vi "Throwing Arm.vi"() -> ()   [LabVIEW 2014]
uses:
  <vilib>/National Instruments/NI Dynamixel API/Dynamixel Driver/Controls/Baud Rate Selector.ctl
  <vilib>/National Instruments/NI Dynamixel API/Dynamixel Driver/Controls/Joints.ctl
  <vilib>/National Instruments/NI Dynamixel API/Dynamixel Driver/Controls/Joint.ctl
  <vilib>/National Instruments/NI Dynamixel API/Dynamixel Driver/Dynamixel Driver Code.lvlib
panel:
  in  "JOSH SWING":dbl[][](array[numeric])=[[2000.0, 150.0, 200.0, 0.0, 60.0, 230.0, 0.0, 223.0], [400.0, 200.0, 270.0, 0.0, 60.0, 230.0, 0.0, 223.0], [400.0, 0.0, 30.0, 0.0, 60.0, 230.0, 0.0, 223.0], [750.0, 220.0, 260.0, 0.0, 60.0, 230.0, 0.0, 223.0], [400.0, 220.0, 260.0, 0.0, 60.0, 230.0, 0.0, 150.0], [600.0, 115.0, 70.0, 0.0, 60.0, 115.0, 0.0, 223.0], [200.0, 115.0, 70.0, 0.0, 60.0, 115.0, 0.0, 223.0], [500.0, 115.0, 70.0, 0.0, 60.0, 115.0, 0.0, 223.0]]
  in  "SWING":dbl[][](array[numeric])=[[400.0, 115.0, 70.0, 0.0, 20.0, 250.0, 0.0, 223.0], [400.0, 0.0, 10.0, 0.0, 120.0, 80.0, 0.0, 223.0], [700.0, 175.0, 70.0, 0.0, 20.0, 250.0, 0.0, 223.0], [500.0, 0.0, 10.0, 0.0, 120.0, 80.0, 0.0, 223.0], [50.0, 350.0, 10.0, 0.0, 120.0, 80.0, 0.0, 223.0], [600.0, 220.0, 260.0, 0.0, 30.0, 230.0, 0.0, 223.0], [200.0, 220.0, 260.0, 0.0, 30.0, 230.0, 0.0, 150.0], [500.0, 115.0, 70.0, 0.0, 60.0, 115.0, 0.0, 223.0]]
  in  "Hard Throw  2":dbl[][](array[numeric])=[[400.0, 115.0, 70.0, 0.0, 20.0, 250.0, 0.0, 223.0], [400.0, 0.0, 10.0, 0.0, 120.0, 80.0, 0.0, 223.0], [700.0, 175.0, 70.0, 0.0, 20.0, 250.0, 0.0, 223.0], [500.0, 0.0, 10.0, 0.0, 120.0, 80.0, 0.0, 223.0], [50.0, 350.0, 10.0, 0.0, 120.0, 80.0, 0.0, 223.0], [600.0, 220.0, 260.0, 0.0, 30.0, 230.0, 0.0, 223.0], [200.0, 220.0, 260.0, 0.0, 30.0, 230.0, 0.0, 150.0], [500.0, 115.0, 70.0, 0.0, 60.0, 115.0, 0.0, 223.0]]
  in  "Gripper\nOpen/Close":bool
  in  "THROW!":bool
  in  "Standard Throw":dbl[][](array[numeric])=[[400.0, 115.0, 70.0, 0.0, 20.0, 250.0, 0.0, 223.0], [400.0, 0.0, 10.0, 0.0, 120.0, 80.0, 0.0, 223.0], [700.0, 175.0, 70.0, 0.0, 20.0, 250.0, 0.0, 223.0], [500.0, 0.0, 10.0, 0.0, 120.0, 80.0, 0.0, 223.0], [50.0, 350.0, 10.0, 0.0, 120.0, 80.0, 0.0, 223.0], [600.0, 220.0, 260.0, 0.0, 30.0, 230.0, 0.0, 223.0], [200.0, 220.0, 260.0, 0.0, 30.0, 230.0, 0.0, 150.0], [500.0, 115.0, 70.0, 0.0, 60.0, 115.0, 0.0, 223.0]]
  out "Elbow":dbl(knob) scale=0.0..300.0
  out "Shoulder Angle":dbl(knob) scale=0.0..300.0
  out "All End Positions":T1 {"Goal Position (Degrees)" scale=0.0..300.0}
  in  "VISA Refnum in":refnum<visa-resource-name>="ASRL1::INSTR"
  in  "Baud Rate":T3
  in  "File Path Control":path=path "/Macintosh HD/Users/joshuasullivan/Dropbox/ROCO504/Showcase/RobotTest.ini"
  in  "Stop Button":bool
  # "Time"
  # "Servo1"
  # "Servo2"
  # "Shoulder"
  # "Servo4"
  # "Servo5"
  # "Elbow"
  # "Servo7"
  # "Elbow bend up"
  # "Move whole arm back"
  # "Whole arm forwards w/ elbow swing"
  # "Whole arm back"
  # "Shoulder build up tension"
  # "Arm forwards closed gripper"
  # "Arm forwards open gripper"
  # "Return and wait"
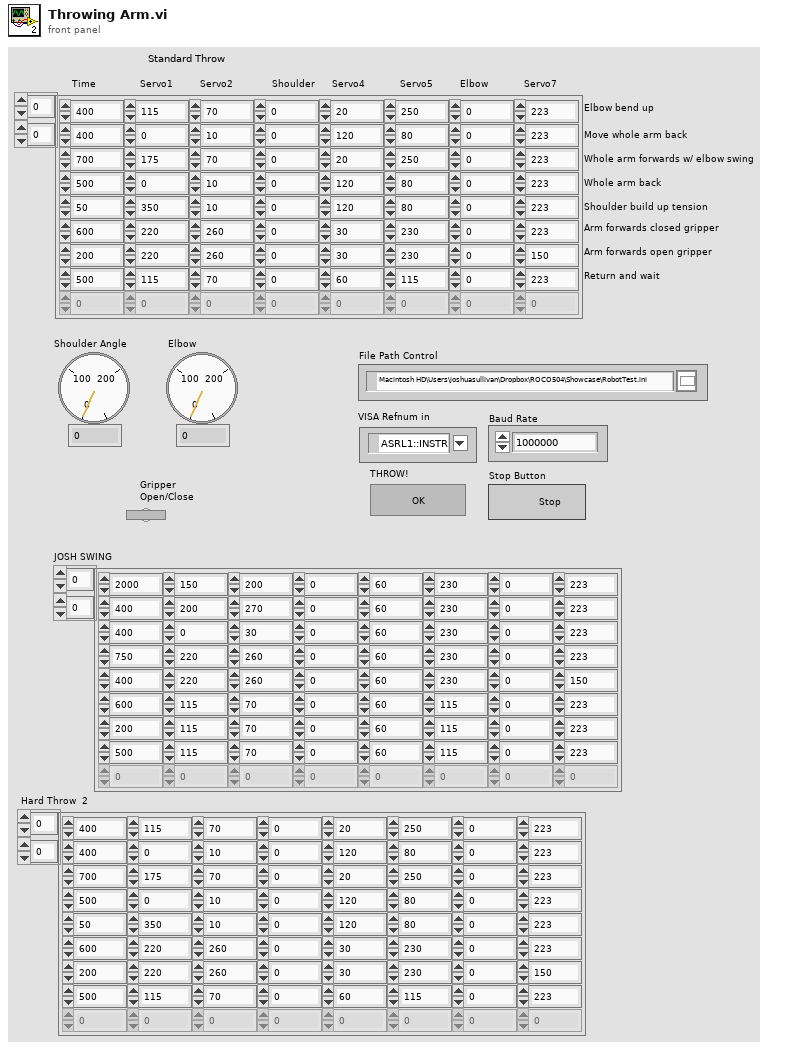
[diagram p1: front panel]
types:
  T1 = typedef "Dynamixel Driver Code.lvlib/Joints.ctl" = T2[]
  T2 = typedef "Dynamixel Driver Code.lvlib/Joint.ctl" = cluster{"Joint ID":dbl, "Goal Position (Degrees)":dbl}
  T3 = typedef "Dynamixel Driver Code.lvlib/Baud Rate Selector.ctl" = enum16{"1000000", "57600"}
  T4 = typedef "Dynamixel Driver Code.lvlib/Dynamixel Data.ctl" = T5[]
  T5 = typedef "Dynamixel Driver Code.lvlib/Single Dynamixel.ctl" = cluster{"ID":u8, "Speed":u16, "CW Margin/D":u8, "CCW Margin/I":u8, "CW Slope/P":u8, "CCW Slope/Accl":u8, "Punch":u16, "Joint":u8, "Max Position (Deg)":u16, "Min Position (Deg)":u16, "Torque Limit":u16, "Motor Type":T6, "Motor Model":T7, "Orientation":T8, "Sync Cable":T9}
  T6 = typedef "Dynamixel Driver Code.lvlib/Master Slave.ctl" = enum16{"Master", "Slave", "Sync"}
  T7 = typedef "Dynamixel Driver Code.lvlib/Motor Model.ctl" = enum16{"AX/DX/RX", "MX", "EX-106+"}
  T8 = typedef "Dynamixel Driver Code.lvlib/Orientation.ctl" = enum16{"Single", "Paired - Opposite", "Paired", "Same ID"}
  T9 = typedef "Dynamixel Driver Code.lvlib/Sync Cable.ctl" = enum16{"No", "Yes"}
  T10 = typedef "Dynamixel Driver Code.lvlib/Robot Session.ctl" = cluster{"VISA Resource":refnum<visa-resource-name>, "Dynamixel Data":T4}
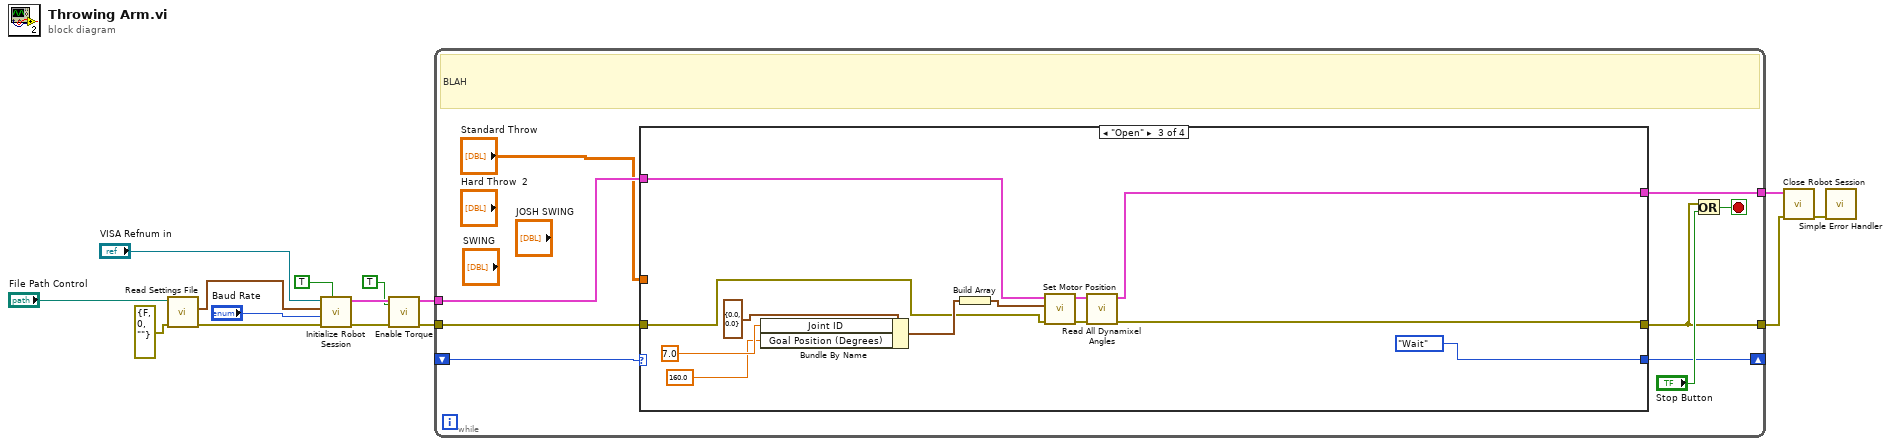
[diagram p0: block diagram]
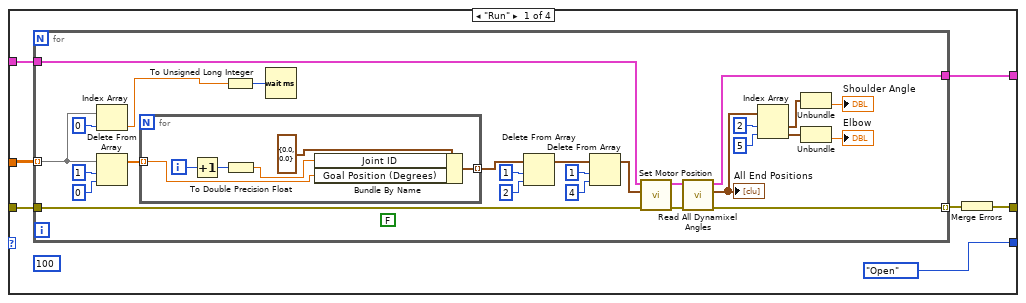
[diagram p2: hidden frame]
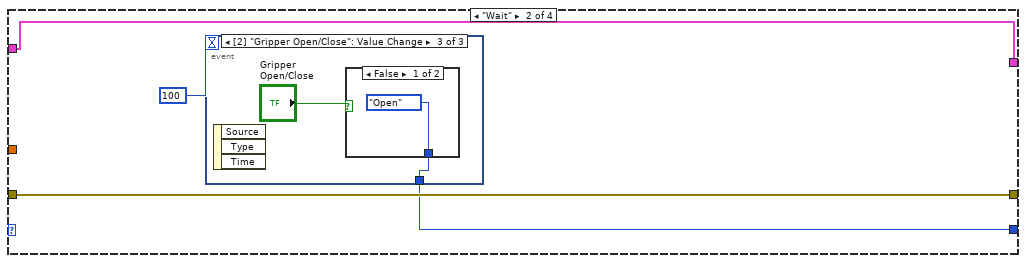
[diagram p3: hidden frame]
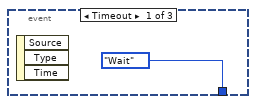
[diagram p4: hidden frame]
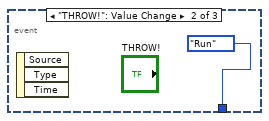
[diagram p5: hidden frame]
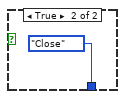
[diagram p6: hidden frame]
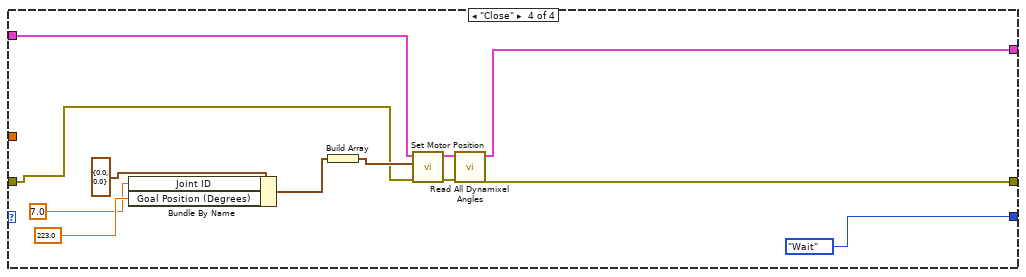
[diagram p7: hidden frame]
diagram:
  n1 = call <vilib>:"Read Settings File.vi"("error in (no error)"=errorcluster {"status"=FALSE, "code"=0, "source"=""} ("error constant"), "file path (dialog if empty)"="File Path Control") -> ("error out"=w14:errorcluster, "Dynamixel Data"=w7:T4)  [unwired: 8 in]
  n2 = call <vilib>:"Initialize Robot Session.vi"("Configure"=TRUE, "error in"=w14, "Baud Rate"="Baud Rate", "Initialization"=w7, "VISA Refnum in"="VISA Refnum in") -> ("error out"=w11:errorcluster, "Robot Session"=w12:T10)  [unwired: 5 in]
  n3 = call <vilib>:"Enable Torque.vi"("Set Goal Position to Current Position before Enable"=TRUE, "error in (no error)"=w11, "Robot Session In"=w12) -> ("error out"=w8:errorcluster, "Robot Session Out"=w10:T10)  [unwired: 6 in, 1 out]
  n4 = while {
    tunnel: w10 -> [w24]
    tunnel: w8 -> [w23]
    tunnel: [w22] -> w3
    tunnel: [w17] -> w2
    shift-right: [w19] -> _
    shift-left: _ -> [w18]
    stop <- w20 stop-if-true
    # "BLAH"
    n5 = case shown="\"Open\"" w18 {
      tunnel: w24 -> [w31 w68 w77 w91]
      tunnel: w23 -> [w30 w67 w76 w88]
      tunnel: [w29 w68 w79 w90] -> w22
      tunnel: [w26 w67 w78 w89] -> w17
      tunnel: "Standard Throw" -> [w28 _ _ _]
      tunnel: [enum16{"Close", "Open", "Wait", "Run"}."Open" w66 enum16{"Close", "Open", "Wait", "Run"}."Wait" enum16{"Close", "Open", "Wait", "Run"}."Wait"] -> w19
      frame "Run" {
        (unwired) 100
        n6 = for {
          tunnel: w28 -> [w54] mode=indexing
          tunnel: w31 -> [w43]
          tunnel: [w42] -> w29
          tunnel: [w41] -> w27 mode=indexing
          tunnel: w30 -> [w40]
          (unwired) FALSE ("stop")
          n7 = Index Array(array=w54, index=0 ("length")) -> (element=w32:dbl)
          n8 = Delete From Array(array=w54, length=1, index=0) -> (array with subset deleted=w55:dbl[])  [unwired: 1 out]
          n9 = for {
            tunnel: w55 -> [w59] mode=indexing
            tunnel: [w60] -> w39 mode=indexing
            i -> [w63]
            n10 = Increment(x=w63) -> (x+1=w62:i32)
            n11 = To Double Precision Float(number=w62) -> (double precision float=w61:dbl)
            n12 = Bundle By Name(cluster=T2 {"Joint ID"=0.0, "Goal Position (Degrees)"=0.0} ("Joint"), "Joint ID"=w61, "Goal Position (Degrees)"=w59) -> (w60:T2)
          }
          n13 = To Unsigned Long Integer(number=w32) -> (unsigned 32bit integer=w53:u32)
          n14 = Wait (ms)(milliseconds to wait=w53) -> ()  [unwired: 1 out]
          n15 = Delete From Array(array=w39, length=1, index=2 ("length")) -> (array with subset deleted=w36:T2[])  [unwired: 1 out]
          n16 = Delete From Array(array=w36, length=1, index=4) -> (array with subset deleted=w35:T2[])  [unwired: 1 out]
          n17 = call <vilib>:"Set Motor Position.vi"("error in (no error)"=w40, "Joints"=w35, "Robot Session In"=w43) -> ("error out"=w52:errorcluster, "Robot Session Out"=w51:T10)  [unwired: 5 in, 2 out]
          n18 = call <vilib>:"Read All Dynamixel Angles.vi"("error in (no error)"=w52, "Robot Session In"=w51) -> ("error out"=w41:errorcluster, "All End Positions"=w50:T1, "Robot Session Out"=w42:T10)  [unwired: 5 in, 2 out]
          "All End Positions" <- w50
          n19 = Index Array(array=w50, index #1=2 ("index"), index #2=5 ("index")) -> (element #1=w47:T2, element #2=w46:T2)
          n20 = Unbundle(w47) -> ("Goal Position (Degrees)"=→"Shoulder Angle":dbl)  [unwired: 1 out]
          n21 = Unbundle(w46) -> ("Goal Position (Degrees)"=→"Elbow":dbl)  [unwired: 1 out]
        }
        n22 = Merge Errors(w27) -> (w26:errorcluster)
      }
      frame "Wait" {
        n23 = event shown="[2] \"Gripper Open/Close\": Value Change" {
          selector: _ -> [_ _ _]
          dyn-events: _ -> [_ _ _]
          timeout: 100 -> [_ _ _]
          tunnel: [enum16{"Close", "Open", "Wait", "Run"}."Wait" enum16{"Close", "Open", "Wait", "Run"}."Run" w71] -> w66
          event Timeout {
            n24 = event-data() -> ()  [unwired: 1 in, 3 out]
          }
          event "THROW!": Value Change {
            n25 = event-data() -> ()  [unwired: 1 in, 3 out]
          }
          event "Gripper\nOpen/Close": Value Change {
            n26 = event-data() -> ()  [unwired: 1 in, 3 out]
            n27 = case shown="False" "Gripper\nOpen/Close" {
              tunnel: [enum16{"Close", "Open", "Wait", "Run"}."Open" enum16{"Close", "Open", "Wait", "Run"}."Close"] -> w71
              frame False {
              }
              frame True {
              }
            }
          }
        }
      }
      frame "Open" {
        n28 = Bundle By Name(cluster=T2 {"Joint ID"=0.0, "Goal Position (Degrees)"=0.0} ("Joint"), "Joint ID"=7.0, "Goal Position (Degrees)"=160.0) -> (w81:T2)
        n29 = Build Array(w81) -> (w80:T2[])
        n30 = call <vilib>:"Set Motor Position.vi"("error in (no error)"=w76, "Joints"=w80, "Robot Session In"=w77) -> ("error out"=w86:errorcluster, "Robot Session Out"=w85:T10)  [unwired: 5 in, 2 out]
        n31 = call <vilib>:"Read All Dynamixel Angles.vi"("error in (no error)"=w86, "Robot Session In"=w85) -> ("error out"=w78:errorcluster, "Robot Session Out"=w79:T10)  [unwired: 5 in, 3 out]
      }
      frame "Close" {
        n32 = Bundle By Name(cluster=T2 {"Joint ID"=0.0, "Goal Position (Degrees)"=0.0} ("Joint"), "Joint ID"=7.0, "Goal Position (Degrees)"=223.0) -> (w97:T2)
        n33 = Build Array(w97) -> (w98:T2[])
        n34 = call <vilib>:"Set Motor Position.vi"("error in (no error)"=w88, "Joints"=w98, "Robot Session In"=w91) -> ("error out"=w92:errorcluster, "Robot Session Out"=w93:T10)  [unwired: 5 in, 2 out]
        n35 = call <vilib>:"Read All Dynamixel Angles.vi"("error in (no error)"=w92, "Robot Session In"=w93) -> ("error out"=w89:errorcluster, "Robot Session Out"=w90:T10)  [unwired: 5 in, 3 out]
      }
    }
    n36 = Or(x=w17, y="Stop Button") -> (x .or. y?=w20:bool)
  }
  n37 = call <vilib>:"Close Robot Session.vi"("error in (no error)"=w2, "Robot Session In"=w3) -> ("error out"=w6:errorcluster)  [unwired: 9 in]
  n38 = call <vilib>:"Simple Error Handler.vi"("error in (no error)"=w6) -> ()  [unwired: 4 in, 5 out]
